vi "PDC_GetDeviceCode.vi"(8 "error in (no error)":errorcluster, 11 "DeviceNo":u32) -> (0 "error out":errorcluster, 2 "ID":u32, 3 "ReturnValue":u32, 4 "ErrorCode":u32)   [LabVIEW 2015]
doc: "This VI retrieves the specified device ID."
uses:
  PDCLIB.dll
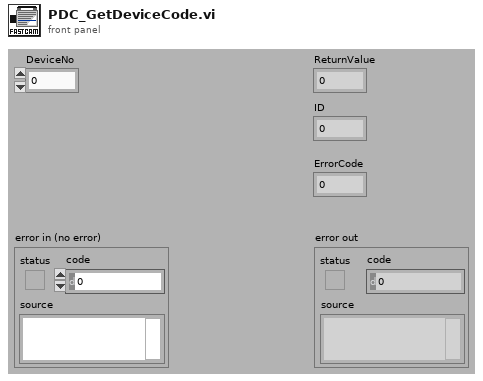
[diagram p1: front panel]
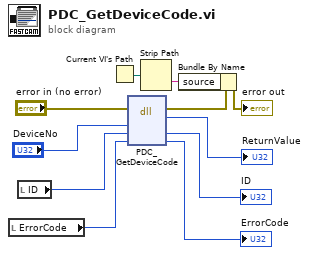
[diagram p0: block diagram]
diagram:
  n1 = local read "ErrorCode"() -> (w8:u32)
  n2 = local read "ID"() -> (w6:u32)
  n3 = Current VI's Path() -> (path=w3:path)
  n4 = dll-call lib="PDCLIB.dll" fn="PDC_GetDeviceCode"(error in="error in (no error)", "nDeviceNo"="DeviceNo", "pCode"=w6, "pErrorCode"=w8) -> (error out=w2:errorcluster, "return type"=→"ReturnValue":u32, "pCode"=→"ID":u32, "pErrorCode"=→"ErrorCode":u32)  [unwired: 3 in, 1 out]
  n5 = Strip Path(path=w3) -> (name=w4:string)  [unwired: 1 out]
  n6 = Bundle By Name(cluster=w2, "source"=w4) -> (→"error out":errorcluster)
